vi "LM35.vi"(8 "Error In":errorcluster, 9 "LINX Resource":T1, 10 "temperatura limite":dbl, 11 "Temperatura optima (led azul)":dbl=0.25 format="%#_13g") -> (0 "Error Out":errorcluster, 1 "LINX Resource 2":T1, 2 "Thermometer":dbl(slide) scale=0.0..100.0, 3 "Color Box 2":u32(colorbox))   [LabVIEW 2018]
uses:
  <vilib>/MakerHub/LINX/Private/Type Defs/LINX Ref.ctl
  <vilib>/MakerHub/LINX/Private/Type Defs/Platform.ctl
  <vilib>/MakerHub/LINX/Private/Type Defs/Interface.ctl
  <vilib>/MakerHub/LINX/Private/Device/Type Defs/LINX Device Config.ctl
  <vilib>/MakerHub/LINX/Private/Device/Type Defs/TCP Config.ctl
  <vilib>/MakerHub/LINX/Private/Device/Type Defs/Channels.ctl
  <vilib>/MakerHub/LINX/Public/Peripherals/PWM/PWM Set Duty Cycle 1 Chan.vi
  <vilib>/MakerHub/LINX/Public/Sensors/Temperature/TMP3x/TMP35.vi
  <vilib>/MakerHub/LINX/Public/Peripherals/PWM/PWM Set Duty Cycle N Chans.vi
  <vilib>/MakerHub/LINX/LMH-LINX.lvlib
  <vilib>/MakerHub/LINX/Public/Sensors/Temperature/TMP3x/TMP3x.lvlib
  <vilib>/ptbypt/NI_PtbyPt.lvlib
  <vilib>/MakerHub/LINX/Private/Device/Device.lvlib
panel:
  in  "intensidd verde":dbl=0.3
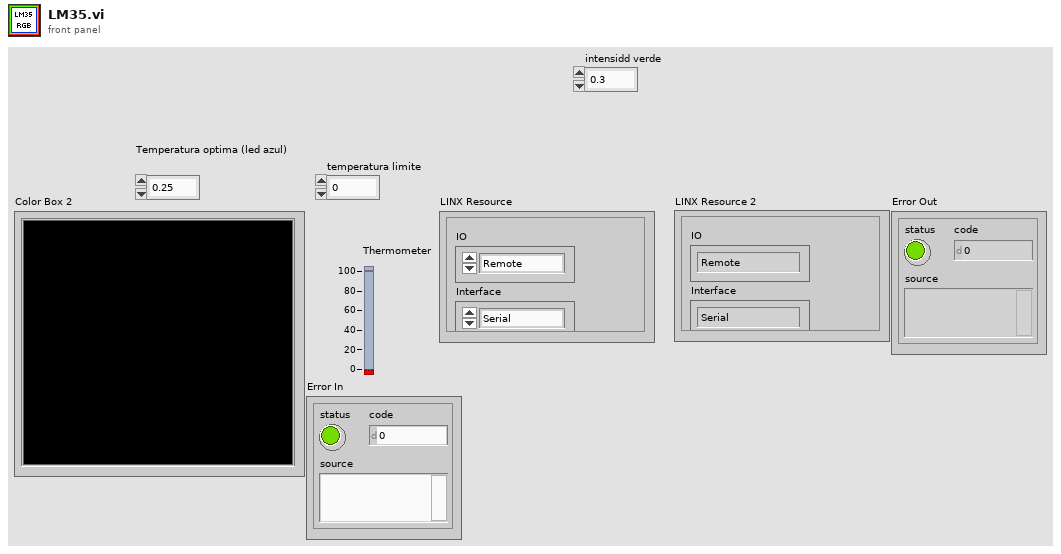
[diagram p1: front panel]
types:
  T1 = typedef "LMH-LINX.lvlib/LINX Ref.ctl" = cluster{"IO":T2, "Interface":T3, "LINX Device Config":T4}
  T2 = typedef "LMH-LINX.lvlib/Platform.ctl" = enum16{"Remote", "Local"}
  T3 = typedef "LMH-LINX.lvlib/Interface.ctl" = enum16{"Serial", "TCP"}
  T4 = typedef "LMH-LINX.lvlib/Device.lvlib/LINX Device Config.ctl" = cluster{"Interface":T3, "COM Port":refnum<visa-resource-name>, "TCP Configuration":T5, "Device Family":u8, "Device ID":u8, "Device Name":string, "TCP Ref":refnum<k5>, "Channels":T6}
  T5 = typedef "LMH-LINX.lvlib/Device.lvlib/TCP Config.ctl" = cluster{"IP Address":string, "Port":u16}
  T6 = typedef "LMH-LINX.lvlib/Channels.ctl" = cluster{"DI":u8[], "DO":u8[], "AI":u8[], "AO":u8[], "PWM":u8[], "QE":u8[], "UART":u8[], "I2C 2":u8[], "SPI":u8[], "CAN":u8[], "Servo":u8[], "AI Ref (V)":dbl, "AI Resolution (Bits)":u8, "AO Ref (V)":dbl, "AO Resolution (Bits)":u8}
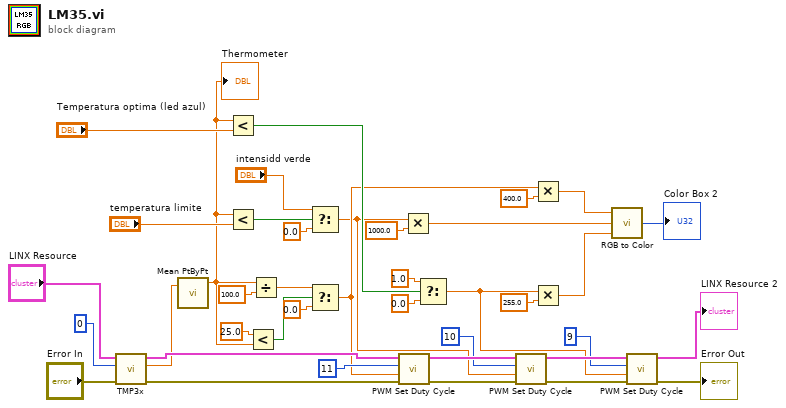
[diagram p0: block diagram]
diagram:
  n1 = call-poly <vilib>:"TMP3x.vi"("Error In"="Error In", "Analog Channel"=u8 0, "LINX Resource"="LINX Resource") -> ("Error Out"=w29:errorcluster, "Temp C"=w11:dbl, "LINX Resource"=w28:T1)  [unwired: 6 in]
  n2 = call <vilib>:"Mean PtByPt.vi"("x"=w11) -> ("mean"=w5:dbl)  [unwired: 3 in, 1 out]
  "Thermometer" <- w5
  n3 = Less?(x=w5, y="Temperatura optima (led azul)") -> (x < y?=w34:bool)
  n4 = Less?(x=w5, y="temperatura limite") -> (x < y?=w10:bool)
  n5 = Less?(x=25.0, y=w5) -> (x < y?=w30:bool)
  n6 = Divide(x=w5, y=100.0) -> (x/y=w25:dbl)
  n7 = Select(t="intensidd verde", s=w10, f=0.0) -> (s? t:f=w9:dbl)
  n8 = Select(t=w25, s=w30, f=0.0) -> (s? t:f=w20:dbl)
  n9 = call-poly <vilib>:"PWM Set Duty Cycle.vi"("Error In"=w29, "Duty Cycle (0-1)"=w20, "PWM Channel"=u32 11, "LINX Resource"=w28) -> ("Error Out"=w38:errorcluster, "LINX Resource"=w39:T1)  [unwired: 6 in]
  n10 = Multiply(x=w9, y=1000.0) -> (x*y=w14:dbl)
  n11 = Select(t=1.0, s=w34, f=0.0) -> (s? t:f=w12:dbl)
  n12 = call-poly <vilib>:"PWM Set Duty Cycle.vi"("Error In"=w38, "Duty Cycle (0-1)"=w9, "PWM Channel"=u8 10, "LINX Resource"=w39) -> ("Error Out"=w36:errorcluster, "LINX Resource"=w37:T1)  [unwired: 6 in]
  n13 = Multiply(x=w20, y=400.0) -> (x*y=w15:dbl)
  n14 = Multiply(x=w12, y=255.0) -> (x*y=w17:dbl)
  n15 = call <vilib>:"RGB to Color.vi"("B"=w17, "G"=w14, "R"=w15) -> ("Color"=→"Color Box 2":u32)
  n16 = call-poly <vilib>:"PWM Set Duty Cycle.vi"("Error In"=w36, "Duty Cycle (0-1)"=w12, "PWM Channel"=u8 9, "LINX Resource"=w37) -> ("Error Out"=→"Error Out":errorcluster, "LINX Resource"=→"LINX Resource 2":T1)  [unwired: 6 in]
